vi "StateActuators.vi"   [LabVIEW 2020]
doc: "This VI performs all of the calculations and decisions related to the swerve drive."
uses:
  GlobalDriverStationCommands.vi
types:
  T1 = enum16{"Off", "Slider", "D_LT", "D_RT", "D_LB", "D_RB", "D_Y", "D_X", "D_A", "D_B", "M_LJoystick", "M_RJoystick", "M_LT", "M_RT", "M_LB", "M_RB", "M_Y", "M_X", "M_A", "M_B"}[]
  T2 = enum16{"Off", "Slider", "D_LT", "D_RT", "D_LB", "D_RB", "D_Y", "D_X", "D_A", "D_B", "M_LJoystick", "M_RJoystick", "M_LT", "M_RT", "M_LB", "M_RB", "M_Y", "M_X", "M_A", "M_B"}
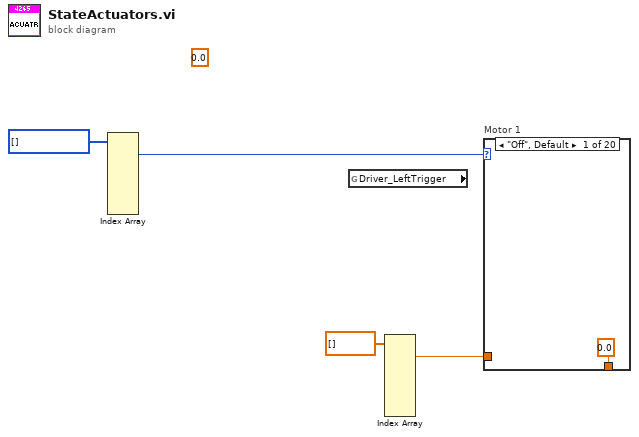
[diagram p0: block diagram]
diagram:
  (unwired) 0.0
  w2 = T1 [] items=["Off", "Slider", "D_LT", "D_RT", "D_LB", "D_RB", "D_Y", "D_X", "D_A", "D_B", "M_LJoystick", "M_RJoystick", "M_LT", "M_RT", "M_LB", "M_RB", "M_Y", "M_X", "M_A", "M_B"] ("array")
  n1 = Index Array(array=w2) -> (element #1=w1:T2)  [unwired: 8 in, 7 out]
  n2 = global read "GlobalDriverStationCommands.vi" "Driver_LeftTrigger"() -> ()  [unwired: 1 out]
  n3 = Index Array(array=dbl[] []) -> (element #1=w3:dbl)  [unwired: 8 in, 7 out]
  n4 = case "Motor 1" shown="\"Off\", Default" w1 {
    tunnel: [0.0 w6 _ _ _ _ _ _ _ _ _ _ _ _ _ _ _ _ _ _] -> _
    tunnel: w3 -> [_ w6 _ _ _ _ _ _ _ _ _ _ _ _ _ _ _ _ _ _]
    frame "Off", Default {
    }
    frame "Slider" {
    }
    frame "D_LT" {
    }
    frame "D_RT" {
    }
    frame "D_LB" {
    }
    frame "D_RB" {
    }
    frame "D_Y" {
    }
    frame "D_X" {
    }
    frame "D_A" {
    }
    frame "D_B" {
    }
    frame "M_LJoystick" {
    }
    frame "M_RJoystick" {
    }
    frame "M_LT" {
    }
    frame "M_RT" {
    }
    frame "M_LB" {
    }
    frame "M_RB" {
    }
    frame "M_Y" {
    }
    frame "M_X" {
    }
    frame "M_A" {
    }
    frame "M_B" {
    }
  }
